vi "OAT LP FIR Design.vi"(8 "A stop [dB]":dbl=72.0 format="%.2f", 9 "stopband":dbl=0.25 format="%.2f", 10 "passband":dbl=0.05 format="%.2f", 11 "fs":dbl=1.0 format="%.2f") -> (0 "error":i32, 3 "filter coefficients":dbl[](array[numeric]) format="%.2f")   [LabVIEW 2017, in "SoundVib_Resampling.lvlib"]
uses:
  <vilib>/addons/Sound and Vibration/Order Analysis/Resample Order Tracking/SoundVib_Resampling.lvlib
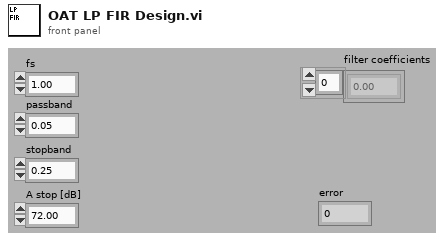
[diagram p1: front panel]
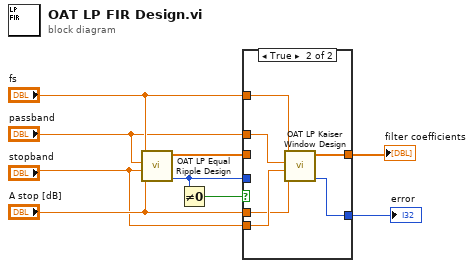
[diagram p0: block diagram]
diagram:
  n1 = call <vilib>:"OAT LP Equal Ripple Design.vi"("A stop [dB]"="A stop [dB]", "stopband"="stopband", "passband"="passband", "fs"="fs") -> ("error"=w5:i32, "filter coefficients"=w3:dbl[])  [unwired: 5 in, 1 out]
  n2 = Not Equal To 0?(x=w5) -> (x != 0?=w4:bool)
  n3 = case shown="True" w4 {
    tunnel: w3 -> [w11 _]
    tunnel: [w11 w12] -> w9
    tunnel: "fs" -> [_ w17]
    tunnel: "passband" -> [_ w16]
    tunnel: "stopband" -> [_ w15]
    tunnel: "A stop [dB]" -> [_ w14]
    tunnel: [w10 w13] -> w6
    tunnel: w5 -> [w10 _]
    frame False {
    }
    frame True {
      n4 = call <vilib>:"OAT LP Kaiser Window Design.vi"("A stop [dB]"=w14, "stopband"=w15, "passband"=w16, "fs"=w17) -> ("error"=w13:i32, "filter coefficients"=w12:dbl[])  [unwired: 5 in, 1 out]
    }
  }
  "filter coefficients" <- w9
  "error" <- w6
